vi "CRYFlatten Virtual Data.vi"(11 "Virtual cluster":T1) -> (3 "Flat Virtual Settings":string)   [LabVIEW 2013]
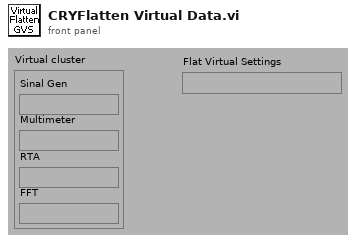
[diagram p1: front panel]
types:
  T1 = cluster{"Sinal Gen":string, "Multimeter":string, "RTA":string, "FFT":string}
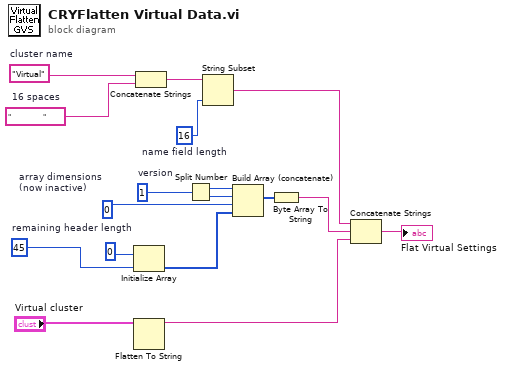
[diagram p0: block diagram]
diagram:
  w4 = u8 0  # array dimensions (now inactive)
  w7 = 16  # name field length
  w8 = "                "  # 16 spaces
  w9 = "Virtual"  # cluster name
  w13 = 45  # remaining header length
  w17 = u16 1  # version
  n1 = Initialize Array(u8 0, w13) -> (w10:u8[])
  n2 = Flatten To String(anything="Virtual cluster") -> (data string=w3:string)  [unwired: 1 in, 4 out]
  n3 = Concatenate Strings(w9, w8) -> (w6:string)
  n4 = Split Number(x=w17) -> (hi(x)=w16:u8, lo(x)=w15:u8)
  n5 = String Subset(string=w6, length (rest)=w7) -> (substring=w5:string)  [unwired: 1 out]
  n6 = Build Array (concatenate)(w16, w15, w4, w10) -> (w12:u8[])
  n7 = Byte Array To String(unsigned byte array=w12) -> (string=w11:string)
  n8 = Concatenate Strings(w5, w11, w3) -> (→"Flat Virtual Settings":string)
